vi "Event Handler Implementation.vi"(8 "error in (no error)":errorcluster, 11 "App in":refnum<class "App.lvclass">) -> (0 "error out":errorcluster, 2 "EventHandlerTask":refnum<class "EventHandlerTask.lvclass">, 3 "App out":refnum<class "App.lvclass">)   [LabVIEW 2020, in "Volatus.lvlib" / "App.lvclass"]
uses:
  App.lvclass
  EventHandlerTask/EventHandlerTask.lvclass
  BasicEventLogger/BasicEventLogger.lvclass
  C:/dev/lv20CE/relink/lv-volatus/Volatus/EventHandlerTask/EventHandlerTask.lvclass
  App.lvclass/App.ctl
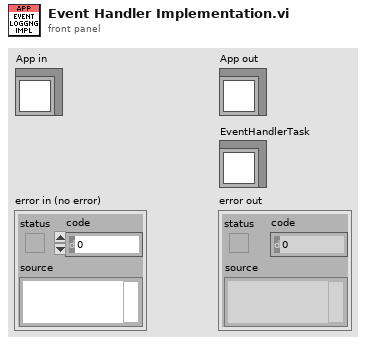
[diagram p1: front panel]
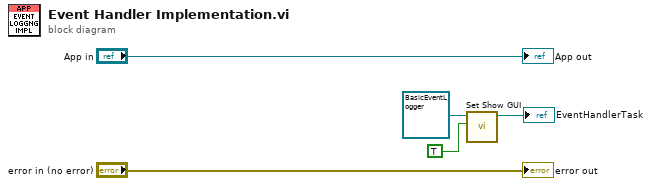
[diagram p0: block diagram]
diagram:
  n1 = call "Set Show GUI.vi"("GUI"=TRUE, "BasicEventLogger in"=refnum<class "BasicEventLogger.lvclass"> refnum ("Volatus:BasicEventLogger.lvclass")) -> ("BasicEventLogger out"=→"EventHandlerTask":refnum<class "BasicEventLogger.lvclass">)  [unwired: 8 in, 1 out]
  "error out" <- "error in (no error)"
  "App out" <- "App in"
